vi "oa_Get DSA 9234 Oversample Rate and Filter Delay.vi"(11 "set sample rate":dbl) -> (0 "input delay":dbl, 1 "SampClkTimebase":dbl, 2 "Actual Sample Rate":dbl)   [LabVIEW 2017, in "SoundVib_TachProcess.lvlib"]
uses:
  <vilib>/addons/Sound and Vibration/Order Analysis/Tach Process/SoundVib_TachProcess.lvlib
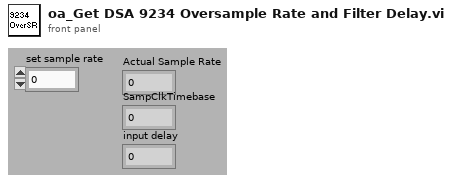
[diagram p1: front panel]
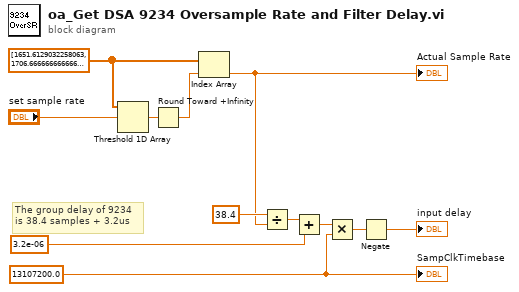
[diagram p0: block diagram]
diagram:
  w2 = 13107200.0 ("SampClkTimebase")
  w9 = dbl[] [1651.6129032258063, 1706.6666666666667, 1765.5172413793102, 1828.5714285714287, 1896.2962962962963, 1969.2307692307693, 2048.0, 2133.3333333333335, 2226.086956521739, 2327.2727272727275, 2438.095238095238, 2560.0, 2694.7368421052633, 2844.4444444444443, 3011.764705882353, 3200.0, 3413.3333333333335, 3657.1428571428573, 3938.4615384615386, 4266.666666666667, 4654.545454545455, 5120.0, 5688.888888888889, 6400.0, 7314.285714285715, 8533.333333333334, 10240.0, 12800.0, 17066.666666666668, 25600.0, 51200.0] ("Array")
  # "The group delay of 9234\nis 38.4 samples + 3.2us"
  n1 = Threshold 1D Array(2:"set sample rate", 3:w9) -> (0:w10:dbl)  [unwired: 1 in]
  n2 = Round Toward +Infinity(x=w10) -> (ceil(x): smallest int >= x=w11:dbl)
  n3 = Index Array(array=w9, index=w11) -> (element=w4:dbl)
  "Actual Sample Rate" <- w4
  n4 = Divide(x=38.4 ("y"), y=w4) -> (x/y=w6:dbl)
  n5 = Add(x=w6, y=3.2e-06) -> (x+y=w8:dbl)
  n6 = Multiply(x=w8, y=w2) -> (x*y=w5:dbl)
  n7 = Negate(x=w5) -> (-x=→"input delay":dbl)
  "SampClkTimebase" <- w2
